vi "Util Convert From Base64.vi"(8 "error in (no error)":errorcluster, 11 "Base64 String":string) -> (0 "error out":errorcluster, 3 "String":string)   [LabVIEW 2010, in "chaosui-crest.lvlib"]
doc: "This VI converts a Base 64 string to its string equivalent. Base64 strings are commonly used in Internet protocols such as HTTP, SMTP, etc."
uses:
  chaosui-crest.lvlib
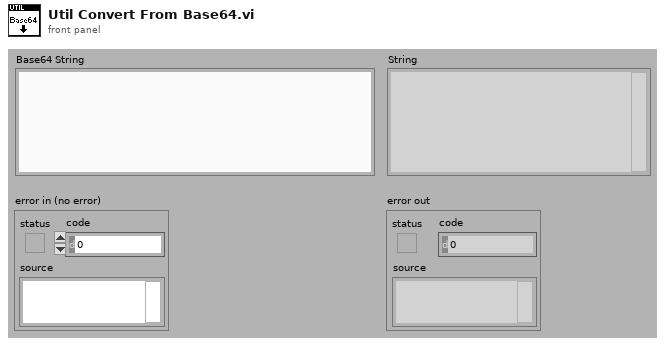
[diagram p1: front panel]
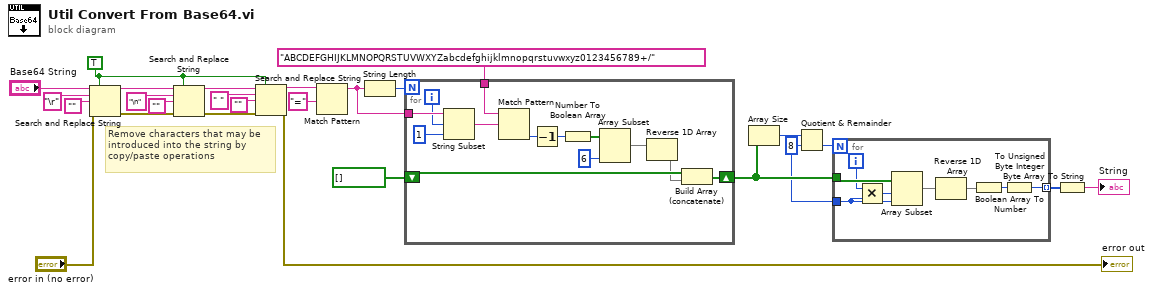
[diagram p0: block diagram]
diagram:
  w1 = TRUE ("replace all? (F)")
  w18 = 8 ("y")
  # "Remove characters that may be\nintroduced into the string by\ncopy/paste operations"
  n1 = Search and Replace String(replace all?=w1, input string="Base64 String", search string="\r" ("replace string (\"\")"), replace string="", error in="error in (no error)") -> (result string=w11:string, error out=w9:errorcluster)  [unwired: 5 out]
  n2 = Search and Replace String(replace all?=w1, input string=w11, search string="\n" ("replace string (\"\")"), replace string="", error in=w9) -> (result string=w5:string, error out=w4:errorcluster)  [unwired: 5 out]
  n3 = Search and Replace String(replace all?=w1, input string=w5, search string=" " ("replace string (\"\")"), replace string="", error in=w4) -> (result string=w2:string, error out=→"error out":errorcluster)  [unwired: 5 out]
  n4 = Match Pattern(string=w2, regular expression="=") -> (before substring=w23:string)  [unwired: 4 out]
  n5 = String Length(string=w23) -> (length=w26:i32)
  n6 = for {
    N: w26 -> [_]
    tunnel: w23 -> [w39]
    tunnel: "ABCDEFGHIJKLMNOPQRSTUVWXYZabcdefghijklmnopqrstuvwxyz0123456789+/" -> [w36]
    shift-right: [w29] -> w19
    shift-left: bool[] [] -> [w28]
    i -> [w37]
    n7 = String Subset(string=w39, offset (0)=w37, length (rest)=1 ("length (rest)")) -> (substring=w35:string)
    n8 = Match Pattern(string=w36, regular expression=w35) -> (offset past match=w34:i32)  [unwired: 1 in, 3 out]
    n9 = Decrement(x=w34) -> (x-1=w33:i32)
    n10 = Number To Boolean Array(number=w33) -> (Boolean array=w32:bool[])
    n11 = Array Subset(array=w32, length=6) -> (w30:bool[])  [unwired: 1 in]
    n12 = Reverse 1D Array(array=w30) -> (reversed array=w27:bool[])
    n13 = Build Array (concatenate)(w28, w27) -> (w29:bool[])
  }
  n14 = Array Size(array=w19) -> (size(s)=w21:i32)
  n15 = Quotient & Remainder(x=w21, y=w18) -> (floor(x/y)=w20:i32)  [unwired: 1 out]
  n16 = for {
    N: w20 -> [_]
    tunnel: w19 -> [w47]
    tunnel: w18 -> [w46]
    tunnel: [w42] -> w17 mode=indexing
    i -> [w45]
    n17 = Multiply(x=w45, y=w46) -> (x*y=w40:i32)
    n18 = Array Subset(array=w47, index=w40, length=w46) -> (w44:bool[])
    n19 = Reverse 1D Array(array=w44) -> (reversed array=w41:bool[])
    n20 = Boolean Array To Number(Boolean array=w41) -> (number=w43:u32)
    n21 = To Unsigned Byte Integer(number=w43) -> (unsigned 8bit integer=w42:u8)
  }
  n22 = Byte Array To String(unsigned byte array=w17) -> (string=→"String":string)
